vi "ExitApplication Event Callback.vi"(4 "Quit Application Event Reference":refnum<user-event>, 6 "CtlRef":refnum<k7>, 7 "Event common data":cluster{"Source":i32, "Type":u32, "Time":u32}) -> ()   [LabVIEW 2010, in "TS Simple LabVIEW OI Dependencies.lvlib"]
uses:
  TS Simple LabVIEW OI Dependencies.lvlib
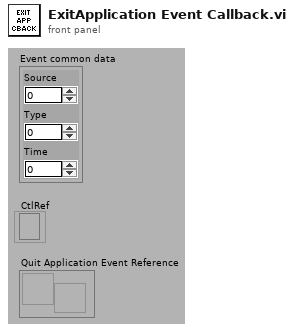
[diagram p1: front panel]
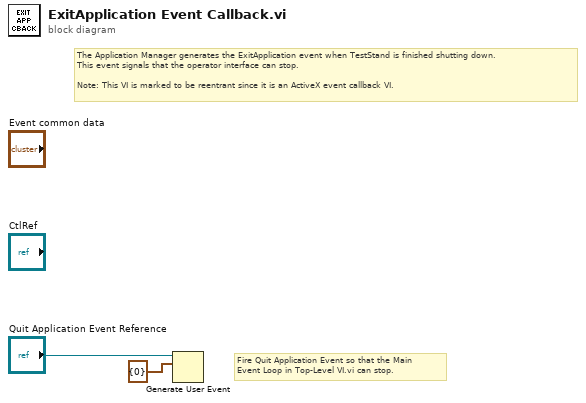
[diagram p0: block diagram]
diagram:
  # "Fire Quit Application Event so that the Main\nEvent Loop in Top-Level VI.vi can stop."
  # "The Application Manager generates the ExitApplication event when TestStand is finished shutting down.\nThis event signals that the operator interface can stop.\n\nNote: This VI is marked to be reentrant since it is an ActiveX event callback VI."
  n1 = Generate User Event(user event="Quit Application Event Reference", event data cluster=cluster{i32} {0}) -> ()  [unwired: 1 in, 2 out]
